vi "Test_LongDelay_StopWhileWaiting_StopImmediately.vi"(8 "error in (no error)":errorcluster, 11 "TestCase in":refnum<class "TestMessageCycle.lvclass">) -> (0 "error out":errorcluster, 3 "TestCase out":refnum<class "TestMessageCycle.lvclass">)   [LabVIEW 2017, in "TestMessageCycle.lvclass"]
uses:
  TestMessageCycle.lvclass
  <vilib>/ActorFramework/Message/Message.lvclass
  Source/MessageCycle/MessageCycle.lvclass/MessageCycle.ctl
  <vilib>/ActorFramework/Message Enqueuer/Message Enqueuer.lvclass/Message Enqueuer.ctl
  <vilib>/ActorFramework/Message Enqueuer/Enqueue.vi
  Doubles/ActorCountsMessageCycles/ActorCountsMessageCycles.lvclass
  C:/Program Files (x86)/National Instruments/LabVIEW 2017/vi.lib/ActorFramework/Actor/Actor.lvclass
  Source/MessageCycle/MessageCycle.lvclass
  C:/Program Files (x86)/National Instruments/LabVIEW 2017/vi.lib/ActorFramework/Message/Message.lvclass
  <vilib>/ActorFramework/Stop Msg/Stop Msg.lvclass
  Source/MessageCycle/Launch Deferred Timeout Notifier.vi
  <vilib>/ActorFramework/Message Priority Queue/Priority Enqueue.vi
  <vilib>/ActorFramework/Actor/Actor.lvclass
panel:
  out "Seconds to stop":dbl
  out "Cyclic Messages Received":u32
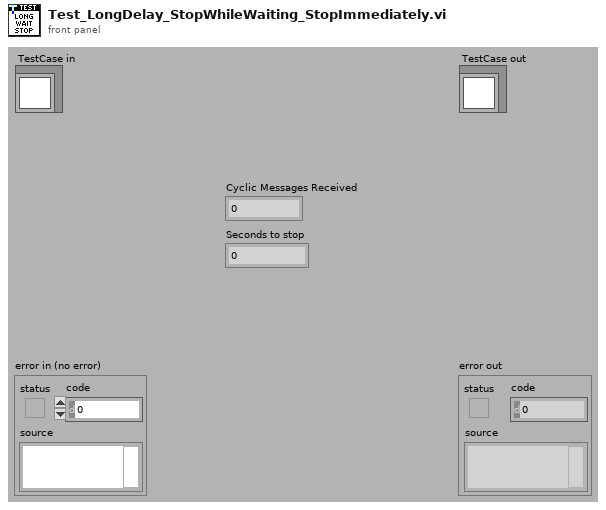
[diagram p1: front panel]
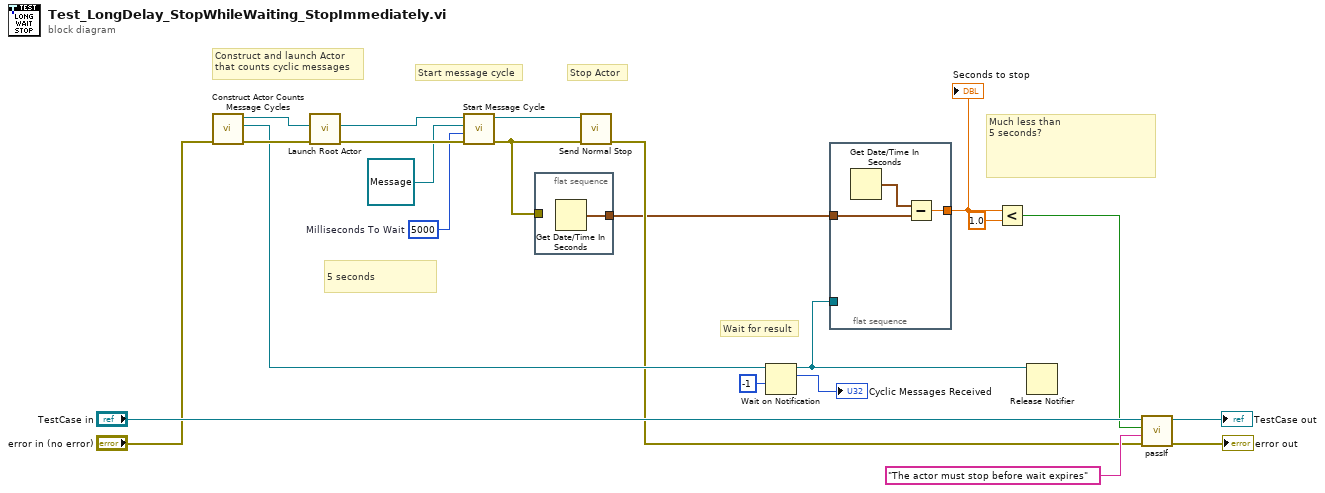
[diagram p0: block diagram]
diagram:
  w17 = 5000  # Milliseconds To Wait
  # "Much less than\n5 seconds?"
  # "5 seconds"
  # "Wait for result"
  # "Stop Actor"
  # "Start message cycle"
  # "Construct and launch Actor\nthat counts cyclic messages"
  n1 = call "Construct Actor Counts Message Cycles.vi"("error in (no error)"="error in (no error)") -> ("error out"=w13:errorcluster, "Final Count"=w12:refnum<notifier>, "ActorCountsMessageCycles"=w14:refnum<class "ActorCountsMessageCycles.lvclass">)  [unwired: 8 in]
  n2 = call <vilib>:"Launch Root Actor.vi"("error in (no error)"=w13, "Actor"=w14) -> ("error out"=w18:errorcluster, "Actor's Enqueuer"=w16:refnum<class "Message Enqueuer.lvclass">)  [unwired: 8 in]
  n3 = call "Start Message Cycle.vi"("error in (no error)"=w18, "Inter-Message Wait [ms] (0)"=w17, "Message"=refnum<class "Message.lvclass"> refnum, "Message Enqueuer"=w16) -> ("error out"=w7:errorcluster, "Message Enqueuer out"=w15:refnum<class "Message Enqueuer.lvclass">)  [unwired: 5 in, 1 out]
  n4 = flat-sequence {
    tunnel: [w23] -> w5
    tunnel: w7 -> [_]
    frame #0 {
      n5 = Get Date/Time In Seconds() -> (seconds since 1Jan1904=w23:timestamp)
    }
  }
  n6 = call <vilib>:"Send Normal Stop.vi"("error in (no error)"=w7, "Message Enqueuer"=w15) -> ("error out"=w10:errorcluster)  [unwired: 9 in]
  n7 = Wait on Notification(notifier=w12, timeout in ms (-1)=-1) -> (notifier out=w6:refnum<notifier>, notification=→"Cyclic Messages Received":u32)  [unwired: 2 in, 2 out]
  n8 = flat-sequence {
    tunnel: w6 -> [_]
    tunnel: w5 -> [w26]
    tunnel: [w24] -> w4
    frame #0 {
      n9 = Get Date/Time In Seconds() -> (seconds since 1Jan1904=w25:timestamp)
      n10 = Subtract(x=w25, y=w26) -> (x-y=w24:dbl)
    }
  }
  n11 = Less?(x=w4, y=1.0) -> (x < y?=w2:bool)
  n12 = Release Notifier(notifier=w6) -> ()  [unwired: 2 in, 3 out]
  n13 = call-dynamic "passIf.vi"("error in (no error)"=w10, "message (\"\")"="The actor must stop before wait expires" ("message (\"\")"), "pass"=w2, "TestCase in"="TestCase in") -> ("error out"=→"error out":errorcluster, "TestCase out"=→"TestCase out":refnum<class "TestMessageCycle.lvclass">)  [unwired: 6 in]
  "Seconds to stop" <- w4
